vi "GetStagePosition.vi"(8 "error in (no error)":errorcluster, 11 "Microscope":refnum<class "Microscope.lvclass">) -> (0 "error out":errorcluster, 2 "Coords":T1, 3 "Microscope out":refnum<class "Microscope.lvclass">)   [LabVIEW 2013, in "Microscope.lvclass"]
doc: "---------------------------------------------------------------\nJKI State Machine Objects™\nhttp://jki.net/state-machine-objects/\nCopyright (C) 2005-2015, JKI <info@jki.net>\nALL RIGHTS RESERVEDJKI State Machine Objects (SMO) 1.0.0.4\nJKI - JKI\nCopyright (c) 2015, JKI"
uses:
  Microscope.lvclass
  XYStage/XYStage.lvclass
  XYStage/Typedefs/(real)Coords--Cluster.ctl
panel:
  # "For instructions on how to use the JKI State Machine Objects, examples and video tutorials, visit:\nhttp://jki.net/state-machine-objects/\n\nJKI State Machine Objects™\nhttp://jki.net/state-machine-objects/\nCopyright (C) 2005-2015, JKI <info@jki.net>\nALL RIGHTS RESERVED"
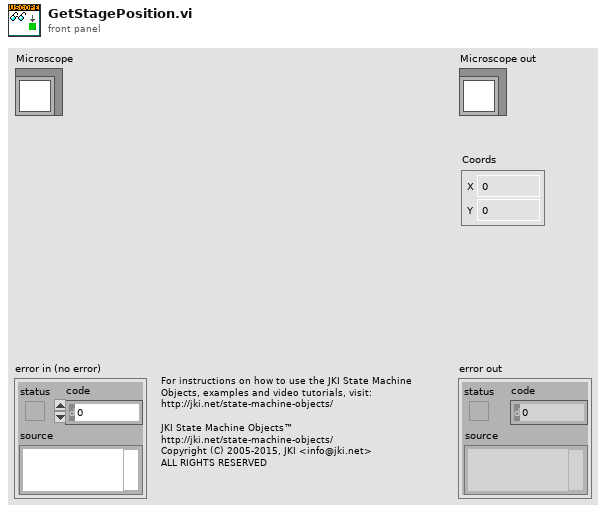
[diagram p1: front panel]
types:
  T1 = typedef "XYStage.lvclass/(real)Coords--Cluster.ctl" = cluster{"X":dbl, "Y":dbl}
  T2 = typedef "Microscope.lvclass/Dependencies--Cluster.ctl" = cluster{"XYStage":refnum<class "XYStage.lvclass">, "Camera":refnum<class "Camera.lvclass">}
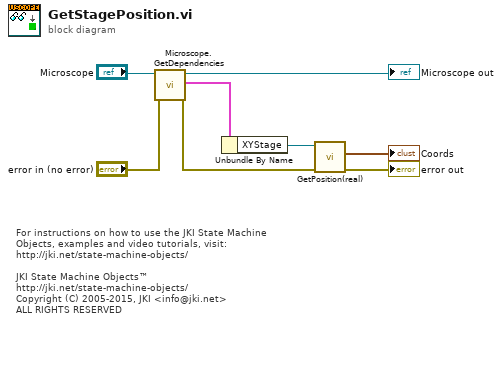
[diagram p0: block diagram]
diagram:
  # "For instructions on how to use the JKI State Machine Objects, examples and video tutorials, visit:\nhttp://jki.net/state-machine-objects/\n\nJKI State Machine Objects™\nhttp://jki.net/state-machine-objects/\nCopyright (C) 2005-2015, JKI <info@jki.net>\nALL RIGHTS RESERVED"
  n1 = call "Microscope.GetDependencies.vi"("error in (no error)"="error in (no error)", "Microscope"="Microscope") -> ("error out"=w2:errorcluster, "Dependencies"=w5:T2, "Microscope out"=→"Microscope out":refnum<class "Microscope.lvclass">)  [unwired: 7 in]
  n2 = Unbundle By Name(w5) -> ("XYStage"=w4:refnum<class "XYStage.lvclass">)
  n3 = call "GetPosition(real).vi"("error in (no error)"=w2, "XYStage"=w4) -> ("error out"=→"error out":errorcluster, "Position"=→"Coords":T1)  [unwired: 7 in, 1 out]
